vi "Fecha y Hora.vi"(11 "Fecha":timestamp) -> (2 "Hora":i32, 3 "Dia":i32)   [LabVIEW 2019, in "Firebase.lvclass"]
uses:
  Firebase.lvclass
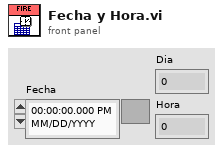
[diagram p1: front panel]
types:
  T1 = typedef "LVDateTimeRec.ctl" = cluster{"fractional second":dbl, "second":i32, "minute":i32, "hour":i32, "day of month":i32, "month":i32, "year":i32, "day of week":i32, "day of year":i32, "DST":i32}
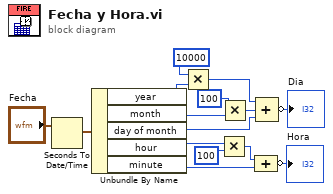
[diagram p0: block diagram]
diagram:
  n1 = Seconds To Date/Time(time stamp (now)="Fecha") -> (date time rec=w14:T1)  [unwired: 1 in]
  n2 = Unbundle By Name(w14) -> ("year"=w13:i32, "month"=w11:i32, "day of month"=w7:i32, "hour"=w5:i32, "minute"=w3:i32)
  n3 = Multiply(x=10000, y=w13) -> (x*y=w8:i32)
  n4 = Multiply(x=w5, y=100 ("x")) -> (x*y=w4:i32)
  n5 = Multiply(x=100, y=w11) -> (x*y=w9:i32)
  n6 = Compound Arithmetic op=ADD(w4, w3) -> (invert →"Hora":i32)
  n7 = Compound Arithmetic op=ADD(w8, w9, w7) -> (invert →"Dia":i32)
